vi "AG Significant Figures.vi"(1 "Number":dbl) -> (0 "Sig Figs":i32)   [LabVIEW 2012]
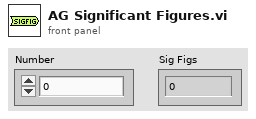
[diagram p1: front panel]
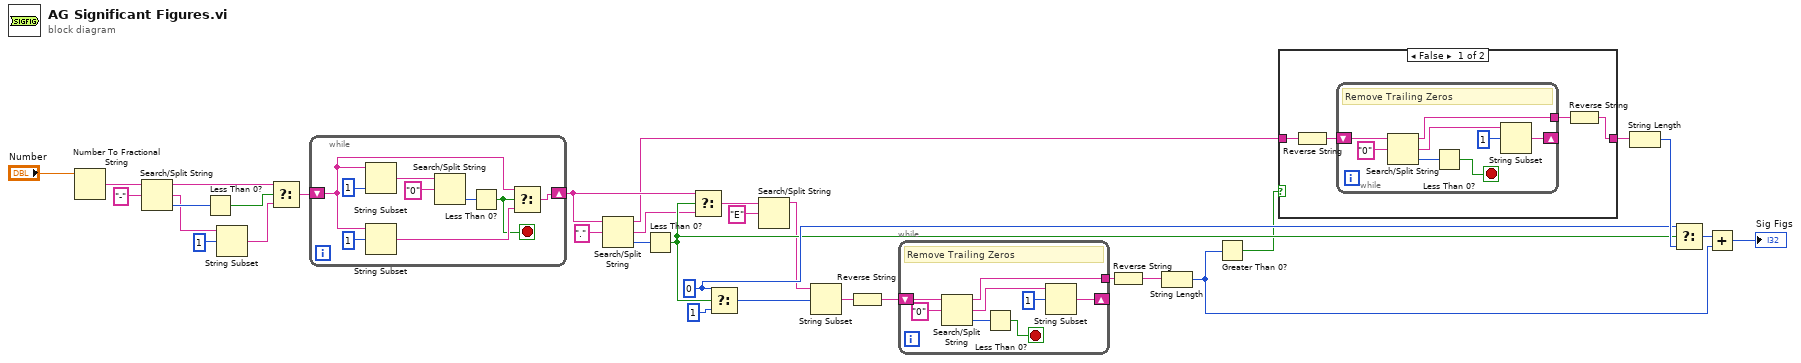
[diagram p0: block diagram]
diagram:
  w25 = 0 ("t")
  n1 = Number To Fractional String(number="Number") -> (F-format string=w2:string)  [unwired: 3 in]
  n2 = Search/Split String(string=w2, search string/char (-)="-") -> (substring before match=w19:string, match + rest of string=w18:string, offset of match=w21:i32)  [unwired: 1 in]
  n3 = Less Than 0?(x=w21) -> (x < 0?=w20:bool)
  n4 = String Subset(string=w18, offset (0)=1) -> (substring=w16:string)  [unwired: 1 in]
  n5 = Select(t=w19, s=w20, f=w16) -> (s? t:f=w14:string)
  n6 = while {
    shift-right: [w38] -> w13
    shift-left: w14 -> [w33]
    stop <- w37 stop-if-true
    n7 = String Subset(string=w33, length (rest)=1 ("length (rest)")) -> (substring=w35:string)  [unwired: 1 in]
    n8 = String Subset(string=w33, offset (0)=1) -> (substring=w41:string)  [unwired: 1 in]
    n9 = Search/Split String(string=w35, search string/char (-)="0") -> (offset of match=w39:i32)  [unwired: 1 in, 2 out]
    n10 = Less Than 0?(x=w39) -> (x < 0?=w37:bool)
    n11 = Select(t=w33, s=w37, f=w41) -> (s? t:f=w38:string)
  }
  n12 = Search/Split String(string=w13, search string/char (-)=".") -> (substring before match=w7:string, match + rest of string=w15:string, offset of match=w30:i32)  [unwired: 1 in]
  n13 = Less Than 0?(x=w30) -> (x < 0?=w24:bool)
  n14 = Select(t=w13, s=w24, f=w15) -> (s? t:f=w29:string)
  n15 = Select(t=w25, s=w24, f=1 ("offset (0)")) -> (s? t:f=w23:i32)
  n16 = Search/Split String(string=w29, search string/char (-)="E") -> (substring before match=w12:string)  [unwired: 1 in, 2 out]
  n17 = String Subset(string=w12, offset (0)=w23) -> (substring=w9:string)  [unwired: 1 in]
  n18 = Reverse String(1:w9) -> (0:w11:string)
  n19 = while {
    shift-right: [w46] -> _
    shift-left: w11 -> [w49]
    tunnel: [w42] -> w10
    stop <- w44 stop-if-true
    # "Remove Trailing Zeros"
    n20 = Search/Split String(string=w49, search string/char (-)="0") -> (substring before match=w42:string, match + rest of string=w43:string, offset of match=w45:i32)  [unwired: 1 in]
    n21 = Less Than 0?(x=w45) -> (x < 0?=w44:bool)
    n22 = String Subset(string=w43, offset (0)=1) -> (substring=w46:string)  [unwired: 1 in]
  }
  n23 = Reverse String(1:w10) -> (0:w8:string)
  n24 = String Length(string=w8) -> (length=w6:i32)
  n25 = Greater Than 0?(x=w6) -> (x > 0?=w4:bool)
  n26 = case shown="False" w4 {
    tunnel: w7 -> [w53 w62]
    tunnel: [w50 w62] -> w5
    frame False {
      n27 = Reverse String(1:w53) -> (0:w52:string)
      n28 = while {
        shift-right: [w58] -> _
        shift-left: w52 -> [w61]
        tunnel: [w54] -> w51
        stop <- w56 stop-if-true
        # "Remove Trailing Zeros"
        n29 = Search/Split String(string=w61, search string/char (-)="0") -> (substring before match=w54:string, match + rest of string=w55:string, offset of match=w57:i32)  [unwired: 1 in]
        n30 = Less Than 0?(x=w57) -> (x < 0?=w56:bool)
        n31 = String Subset(string=w55, offset (0)=1) -> (substring=w58:string)  [unwired: 1 in]
      }
      n32 = Reverse String(1:w51) -> (0:w50:string)
    }
    frame True {
    }
  }
  n33 = String Length(string=w5) -> (length=w28:i32)
  n34 = Select(t=w25, s=w24, f=w28) -> (s? t:f=w27:i32)
  n35 = Add(x=w27, y=w6) -> (x+y=→"Sig Figs":i32)
